vi "Test Sinewave Class.vi"(8 "error in":errorcluster, 11 "TestCase in":refnum<class "Test FGEN.lvclass">) -> (0 "error out":errorcluster, 3 "TestCase out":refnum<class "Test FGEN.lvclass">)   [LabVIEW 2020, in "Test FGEN.lvclass"]
uses:
  Test FGEN.lvclass
  Libraries/FGen/Generador/Generador.lvclass
  <vilib>/addons/_JKI Toolkits/VI Tester/TestCase.llb/TestCase.lvclass
  <vilib>/measure/NI_MABase.lvlib
  C:/Program Files (x86)/National Instruments/LabVIEW 2020/vi.lib/addons/_JKI Toolkits/VI Tester/TestCase.llb/TestCase.lvclass
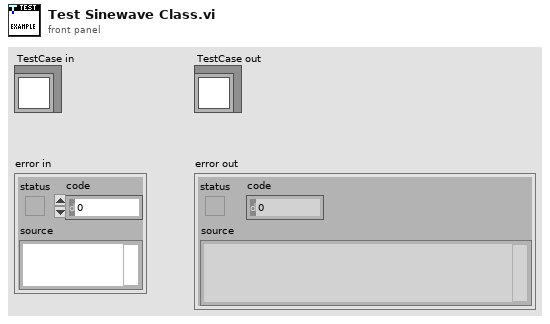
[diagram p1: front panel]
types:
  T1 = enum16{"Sine Wave", "Triangle Wave", "Square Wave", "Sawtooth Wave"}
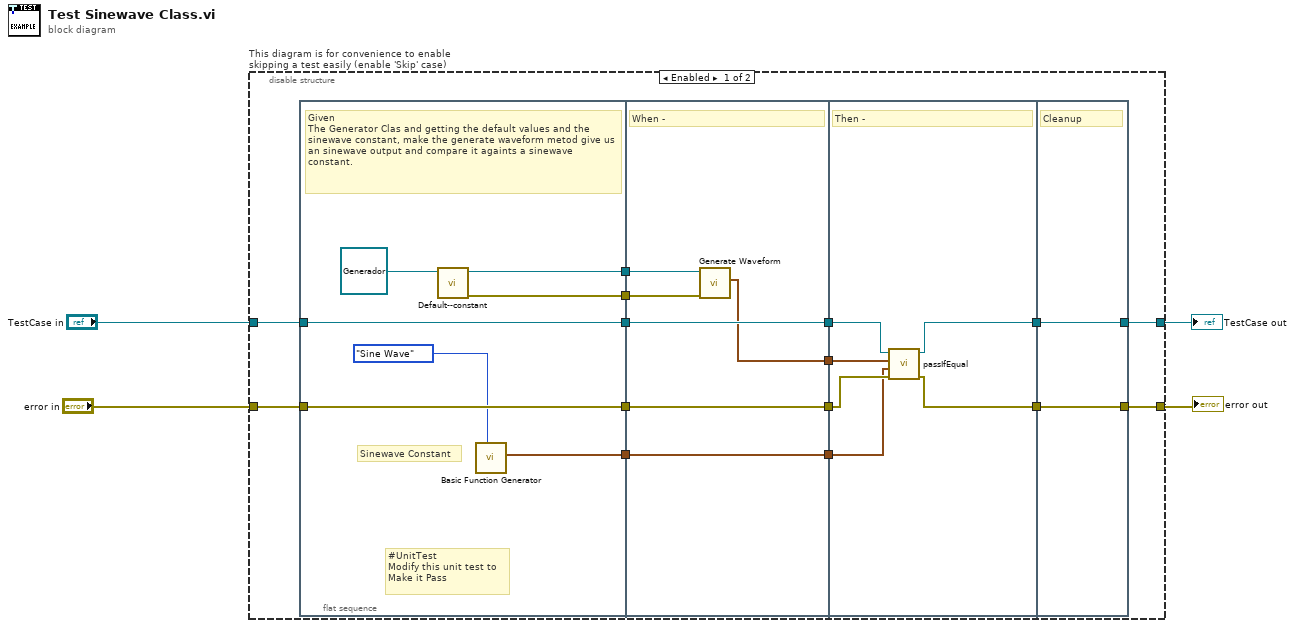
[diagram p0: block diagram]
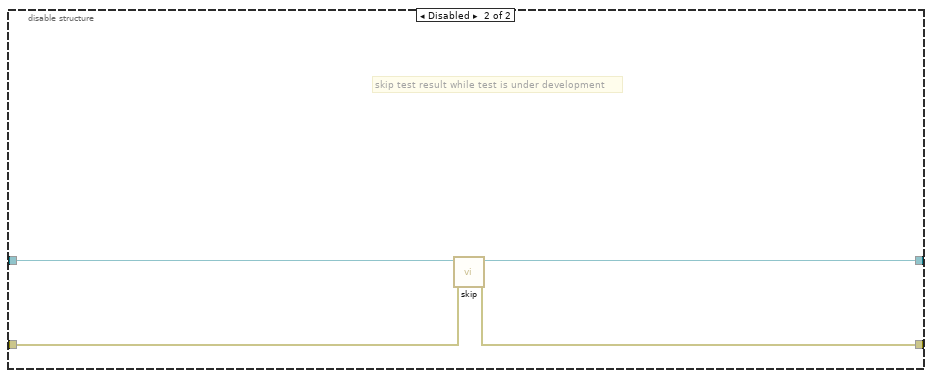
[diagram p2: hidden frame]
diagram:
  n1 = disable-structure "This diagram is for convenience to enable skipping a test easily (enable 'Skip' case)" shown="Enabled" {
    disable-tunnel: "TestCase in" -> [w11 w42]
    disable-tunnel: [w10 w41] -> w1
    disable-tunnel: [w18 w44] -> w3
    disable-tunnel: "error in" -> [w17 w43]
    frame Enabled {
      n2 = flat-sequence {
        tunnel: w11 -> [w25]
        tunnel: [w25] -> w14
        tunnel: w17 -> [w26]
        tunnel: [w26] -> w15
        tunnel: [w23] -> w9
        tunnel: [w22] -> w7
        tunnel: [w21] -> w5
        tunnel: [w31] -> w13
        tunnel: w14 -> [w31]
        tunnel: [w32] -> w16
        tunnel: w15 -> [w32]
        tunnel: w9 -> [w30]
        tunnel: [w29] -> w8
        tunnel: w7 -> [w28]
        tunnel: [w27] -> w6
        tunnel: w5 -> [w27]
        tunnel: [w35] -> w12
        tunnel: [w38] -> w19
        tunnel: w13 -> [w36]
        tunnel: w16 -> [w37]
        tunnel: w8 -> [w34]
        tunnel: w6 -> [w33]
        tunnel: [w40] -> w18
        tunnel: [w39] -> w10
        tunnel: w12 -> [w39]
        tunnel: w19 -> [w40]
        frame #0 {
          # "Sinewave Constant"
          # "#UnitTest\nModify this unit test to\nMake it Pass"
          # "Given\nThe Generator Clas and getting the default values and the sinewave constant, make the generate waveform metod give us an sinewave output and compare it againts a sinewave constant."
          n3 = call-dynamic "Default--constant.vi"("Generator in"=refnum<class "Generador.lvclass"> refnum ("FGen.lvlib:Generator")) -> ("error out"=w22:errorcluster, "Generator out"=w23:refnum<class "Generador.lvclass">)  [unwired: 9 in]
          n4 = call <vilib>:"Basic Function Generator.vi"("signal type"=T1."Sine Wave") -> ("signal out"=w21:waveform(dbl))  [unwired: 8 in, 2 out]
        }
        frame #1 {
          # "When -"
          n5 = call "Generate Waveform.vi"("error in"=w28, "Generator in"=w30) -> ("Waveform"=w29:waveform(dbl))  [unwired: 7 in, 2 out]
        }
        frame #2 {
          # "Then -"
          n6 = call-dynamic "passIfEqual.vi"("error in (no error)"=w37, "y"=w33, "x"=w34, "TestCase in"=w36) -> ("error out"=w38:errorcluster, "TestCase out"=w35:refnum<class "Test FGEN.lvclass">)  [unwired: 6 in]
        }
        frame #3 {
          # "Cleanup"
        }
      }
    }
    frame Disabled {
      # "skip test result while test is under development"
      n7 = call <vilib>:"skip.vi"("error in (no error)"=w43, "TestCase in"=w42) -> ("error out"=w44:errorcluster, "TestCase out"=w41:refnum<class "Test FGEN.lvclass">)  [unwired: 8 in]
    }
  }
  "error out" <- w3
  "TestCase out" <- w1
